vi "Get VI Names.vi"(8 "error in":errorcluster, 11 "VI References":refnum<vi>[](array[refnum])) -> (0 "error out":errorcluster, 3 "Clone Names":string[](array[string]))   [LabVIEW 2014, in "Waveform-Processing-Custom-Device Engine.lvlib" / "Inline Async API.lvlib"]
uses:
  Inline Async API.lvlib
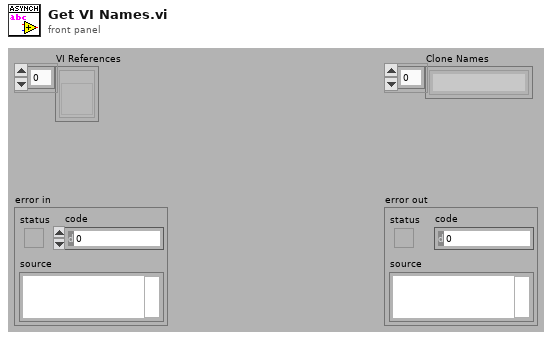
[diagram p1: front panel]
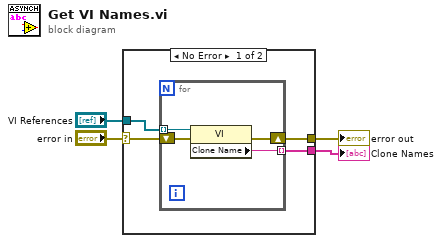
[diagram p0: block diagram]
diagram:
  n1 = case shown="No Error" "error in" {
    selector: "error in" -> [w5 w13]
    tunnel: "VI References" -> [w8 _]
    tunnel: [w7 _] -> w1
    tunnel: [w6 w13] -> w3
    frame No Error {
      n2 = for {
        tunnel: w8 -> [w12] mode=indexing
        tunnel: [w11] -> w7 mode=indexing
        shift-right: [w10] -> w6
        shift-left: w5 -> [w9]
        n3 = property class="VI"(reference=w12, error in=w9) -> (error out=w10:errorcluster, "Clone Name"=w11:string)  [unwired: 1 out]
      }
    }
    frame Error {
    }
  }
  "error out" <- w3
  "Clone Names" <- w1
